vi "Steering Frame Options to Wheel Options.vi"(10 "draw steering frame options":T2={"draw wheel states?"=FALSE, "highlight wheel index"=-1, "pixels per unit"=10.0, "draw forward velocity?"=FALSE, "velocity scale"=1.0}, 11 "draw wheel options in":T1={"global wheel position"={"x"=0.0, "y"=0.0}, "wheel frame angle (rad)"=0.0, "color (black)"=0, "draw wheel state"=FALSE, "draw forward velocity"=FALSE, "velocity scale"=0.0, "velocity color (red)"=16711680}) -> (3 "draw wheel options out":T1={"global wheel position"={"x"=0.0, "y"=0.0}, "wheel frame angle (rad)"=0.0, "color (black)"=0, "draw wheel state"=FALSE, "draw forward velocity"=FALSE, "velocity scale"=0.0, "velocity color (red)"=16711680})   [LabVIEW 2017, in "NI_Robotics_Steering Picture.lvlib"]
uses:
  <vilib>/robotics/Utilities/Visualization/Steering Visualization/Steering Picture/NI_Robotics_Steering Picture.lvlib
  <vilib>/robotics/Utilities/Visualization/Steering Visualization/Steering Picture/Draw Steering Frame Options.ctl
  <vilib>/robotics/Utilities/Visualization/Steering Visualization/Steering Picture/Draw Wheel Options.ctl
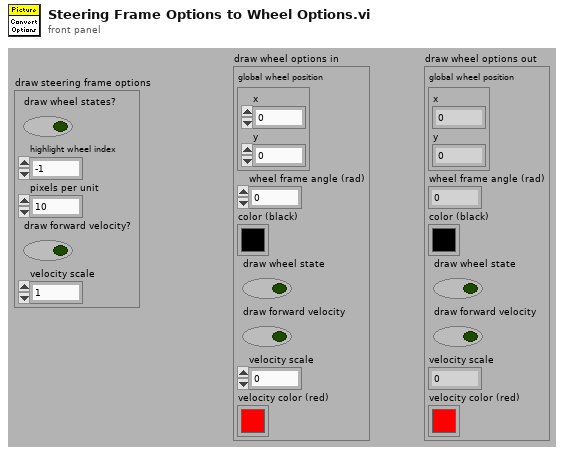
[diagram p1: front panel]
types:
  T1 = typedef "NI_Robotics_Steering Picture.lvlib/Draw Wheel Options.ctl" = cluster{"global wheel position":cluster{"x":dbl, "y":dbl}, "wheel frame angle (rad)":dbl, "color (black)":u32, "draw wheel state":bool, "draw forward velocity":bool, "velocity scale":dbl, "velocity color (red)":u32}
  T2 = typedef "NI_Robotics_Steering Picture.lvlib/Draw Steering Frame Options.ctl" = cluster{"draw wheel states?":bool, "highlight wheel index":i32, "pixels per unit":dbl, "draw forward velocity?":bool, "velocity scale":dbl}
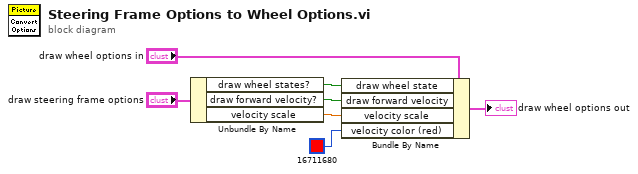
[diagram p0: block diagram]
diagram:
  n1 = Unbundle By Name("draw steering frame options") -> ("draw wheel states?"=w4:bool, "draw forward velocity?"=w1:bool, "velocity scale"=w3:dbl)
  n2 = Bundle By Name(cluster="draw wheel options in", "draw wheel state"=w4, "draw forward velocity"=w1, "velocity scale"=w3, "velocity color (red)"=u32 16711680) -> (→"draw wheel options out":T1)
